vi "Setup UI.vi"(8 "error in (no error)":errorcluster, 10 "Set UI to input? (F)":bool, 11 "Function Gen Scan in":refnum<class "Function Gen Scan.lvclass">) -> (0 "error out":errorcluster, 3 "Function Gen Scan out":refnum<class "Function Gen Scan.lvclass">)   [LabVIEW 2009, in "Function Gen Scan.lvclass"]
doc: "Scanner::Setup is a constructor that has no parameters and faces the user. The Factory calls this VI to let the user configure this Scanner. It is dynamically dispatched in order to let the user choose the type as well as the options of the scanner."
uses:
  Function Gen Scan.lvclass
  Instruments/Function Generator/Tektronix AFG 3000 Series/controls.llb/Channel.ctl
  Function Gen Scan.lvclass/Function Gen Scan.ctl
panel:
  in  "Send conds for first point to FG":bool
  in  "Channel (0: Channel 1)":T1 items=["Channel 1", "Channel 2"]
  in  "Amplitude (Vpp)":dbl[unit]
  # "Function Gen Scan"
  # "Note: Independent Variable \nabove must be given in MHz."
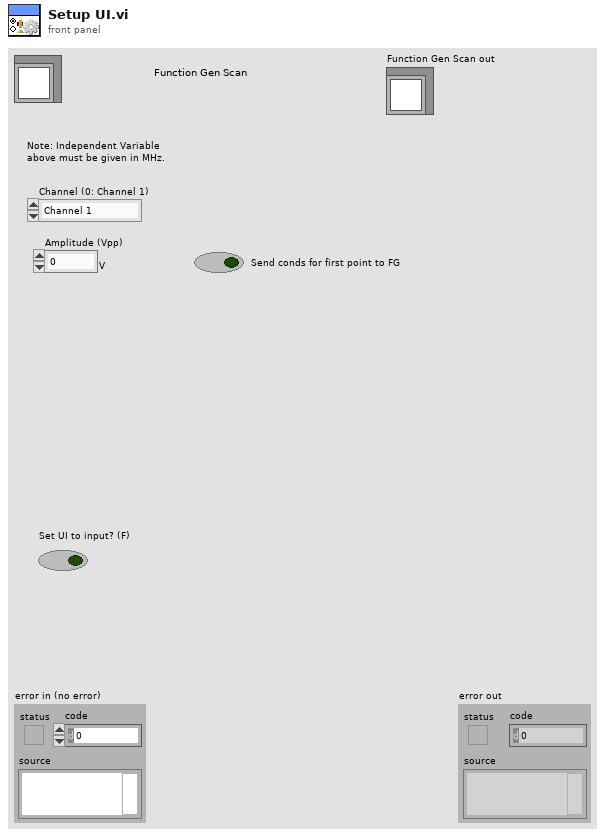
[diagram p1: front panel]
types:
  T1 = typedef "Channel.ctl" = u16
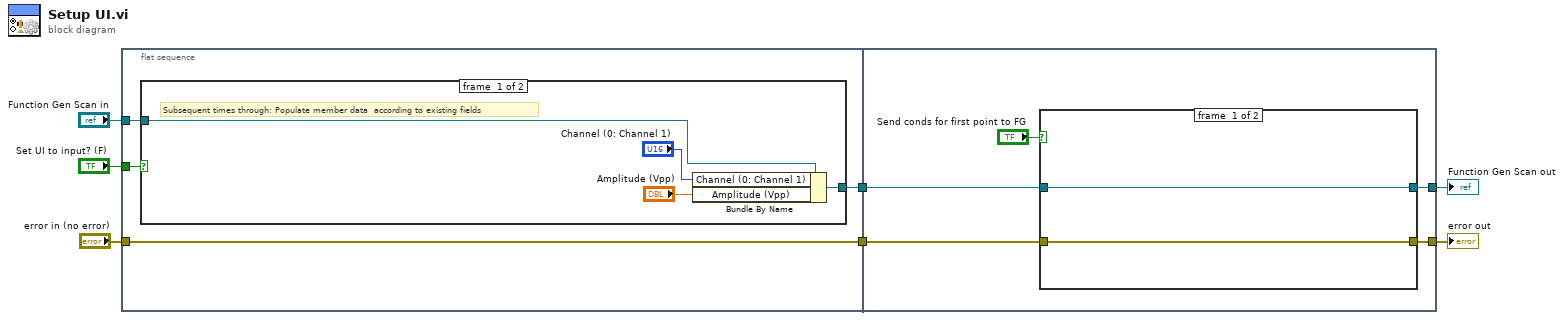
[diagram p0: block diagram]
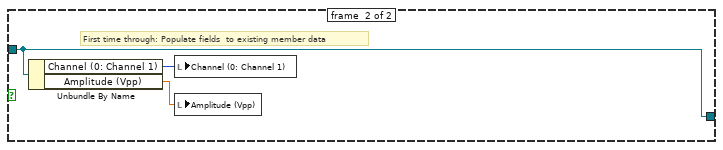
[diagram p2: hidden frame]
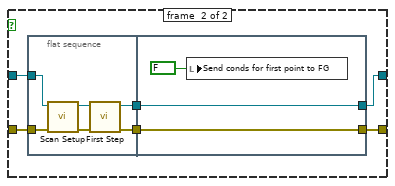
[diagram p3: hidden frame]
diagram:
  n1 = flat-sequence {
    tunnel: "Set UI to input? (F)" -> [w11]
    tunnel: "Function Gen Scan in" -> [w10]
    tunnel: [w9] -> w5
    tunnel: [w8] -> w2
    tunnel: "error in (no error)" -> [w8]
    tunnel: w5 -> [w22]
    tunnel: [w21] -> w4
    tunnel: [w19] -> w3
    tunnel: w2 -> [w20]
    frame #0 {
      n2 = case shown="False" w11 {
        tunnel: w10 -> [w15 w18]
        tunnel: [w12 w18] -> w9
        frame #0 {
          # "Subsequent times through: Populate member data  according to existing fields"
          n3 = Bundle By Name(cluster=w15, "Channel (0: Channel 1)"="Channel (0: Channel 1)", "Amplitude (Vpp)"="Amplitude (Vpp)") -> (w12:refnum<class "Function Gen Scan.lvclass">)
        }
        frame #1 {
          # "First time through: Populate fields  to existing member data"
          n4 = Unbundle By Name(w18) -> ("Channel (0: Channel 1)"=w17:T1, "Amplitude (Vpp)"=w16:dbl[unit])
          n5 = local write "Channel (0: Channel 1)"(w17) -> ()
          n6 = local write "Amplitude (Vpp)"(w16) -> ()
        }
      }
    }
    frame #1 {
      n7 = case shown="True" "Send conds for first point to FG" {
        tunnel: w22 -> [w25 w31]
        tunnel: [w25 w30] -> w21
        tunnel: w20 -> [w24 w29]
        tunnel: [w24 w28] -> w19
        frame #0 {
        }
        frame #1 {
          n8 = flat-sequence {
            tunnel: w31 -> [w37]
            tunnel: w29 -> [w34]
            tunnel: [w35] -> w27
            tunnel: [w32] -> w26
            tunnel: [w39] -> w28
            tunnel: [w40] -> w30
            tunnel: w27 -> [w40]
            tunnel: w26 -> [w39]
            frame #0 {
              n9 = call-dynamic "Scan Setup.vi"("error in (no error)"=w34, "Function Gen Scan in"=w37) -> ("error out"=w33:errorcluster, "Function Gen Scan out"=w36:refnum<class "Function Gen Scan.lvclass">)  [unwired: 8 out]
              n10 = call-dynamic "First Step.vi"("error in (no error)"=w33, "Function Gen Scan.lvclass in"=w36) -> ("error out"=w32:errorcluster, "Function Gen Scan.lvclass out"=w35:refnum<class "Function Gen Scan.lvclass">)  [unwired: 8 out]
            }
            frame #1 {
              n11 = local write "Send conds for first point to FG"(FALSE ("Send conds for first point to FG")) -> ()
            }
          }
        }
      }
    }
  }
  "error out" <- w3
  "Function Gen Scan out" <- w4
